vi "Read User file - copia.vi"(0 "file path (use dialog)":path, 11 "error in":errorcluster) -> (4 "Array":T1[](array[typedef]), 15 "error out":errorcluster)   [LabVIEW 2012]
doc: "This Function is designed to read in a text file and retunr an array of string with each line of the text file. \n\nFor comments or questions about this code please look at the community example page below.\nhttp://decibel.ni.com/content/docs/DOC-10662"
uses:
  typedef/User_Data_Cluster.ctl
  typedef/User Accounts.ctl
panel:
  in  "Array 2":T1[](array[typedef])
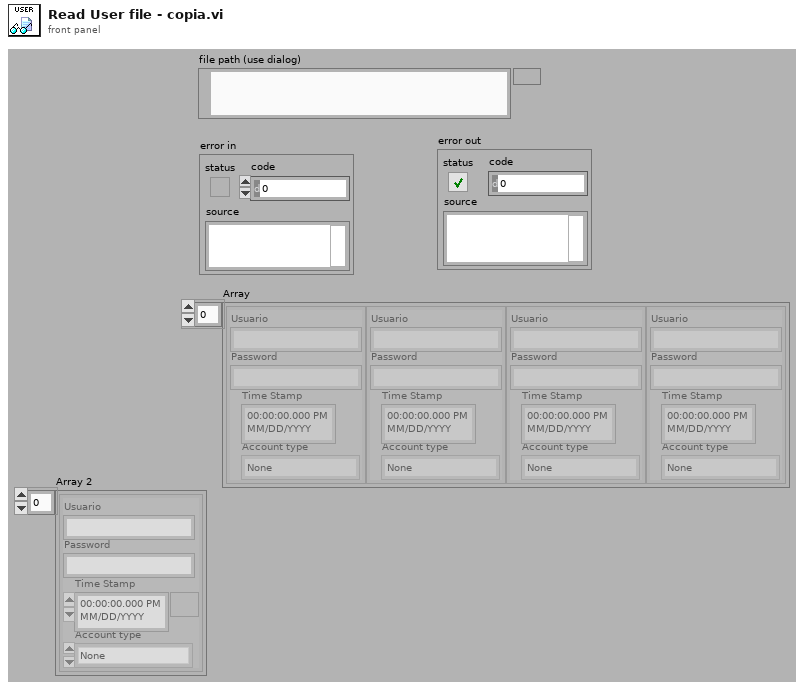
[diagram p1: front panel]
types:
  T1 = typedef "User_Data_Cluster.ctl" = cluster{"Usuario":string, "Password":string, "Account type":T2, "Time Stamp":timestamp}
  T2 = typedef "User Accounts.ctl" = enum16{"None", "User", "Admin"}
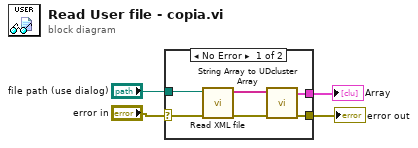
[diagram p0: block diagram]
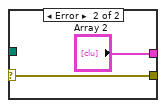
[diagram p2: hidden frame]
diagram:
  n1 = case shown="No Error" "error in" {
    selector: "error in" -> [w5 w12]
    tunnel: "file path (use dialog)" -> [w10 _]
    tunnel: [w8 "Array 2"] -> w3
    tunnel: [w6 w12] -> w2
    frame No Error {
      n2 = call "Read XML file.vi"("error in (no error)"=w5, "file path (use dialog)"=w10) -> ("error out"=w7:errorcluster, "Array 3"=w9:string[])  [unwired: 8 in]
      n3 = call "String Array to UDcluster Array.vi"("error in (no error)"=w7, "Array 3"=w9) -> ("error out"=w6:errorcluster, "Array"=w8:T1[])  [unwired: 8 in]
    }
    frame Error {
    }
  }
  "error out" <- w2
  "Array" <- w3
